vi "fgv_measure_reg.vi"(7 "cmd":T2, 11 "measure_reg":T1) -> (3 "measure_reg 2":T1)   [LabVIEW 2019]
uses:
  _ctrl/rw.ctl
  measure_reg.ctl
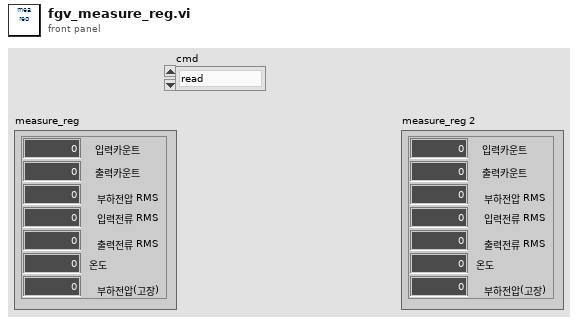
[diagram p1: front panel]
types:
  T1 = typedef "measure_reg.ctl" = cluster{"입력카운트":dbl, "출력카운트":dbl, "부하전압 RMS":dbl, "입력전류 RMS":dbl, "출력전류 RMS":dbl, "온도":dbl, "부하전압(고장)":dbl}
  T2 = typedef "rw.ctl" = enum16{"read", "write"}
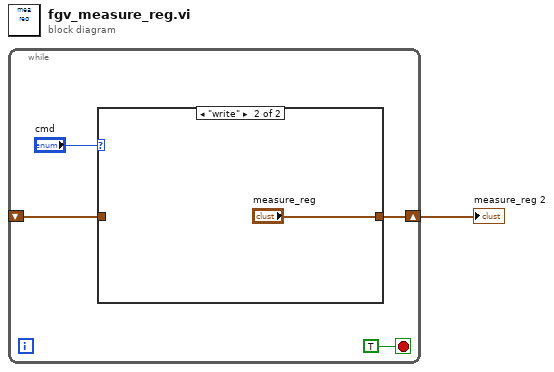
[diagram p0: block diagram]
diagram:
  n1 = while {
    shift-right: [w3] -> w1
    shift-left: _ -> [w2]
    stop <- TRUE stop-if-true
    n2 = case shown="\"write\"" "cmd" {
      tunnel: [w6 "measure_reg"] -> w3
      tunnel: w2 -> [w6 _]
      frame "read", Default {
      }
      frame "write" {
      }
    }
  }
  "measure_reg 2" <- w1
